vi "GetOpenChannels.vi"(7 "Slot":T1, 8 "Error In":errorcluster, 11 "Keithley 7001 In":refnum<visa-resource-name>) -> (0 "Error Out":errorcluster, 2 "Channels Opened?":bool[](array[boolean]), 3 "Keithley 7001 Out":refnum<visa-resource-name>)   [LabVIEW 2012, in "Keithley-7001.lvlib"]
uses:
  Keithley-7001.lvlib
  Controls/Slot.ctl
panel:
  # "33"
  # "34"
  # "35"
  # "1"
  # "2"
  # "3"
  # "4"
  # "5"
  # "6"
  # "7"
  # "8"
  # "9"
  # "10"
  # "11"
  # "12"
  # "13"
  # "14"
  # "15"
  # "16"
  # "17"
  # "18"
  # "19"
  # "20"
  # "21"
  # "22"
  # "23"
  # "24"
  # "25"
  # "26"
  # "27"
  # "28"
  # "29"
  # "30"
  # "31"
  # "32"
  # "36"
  # "37"
  # "38"
  # "39"
  # "40"
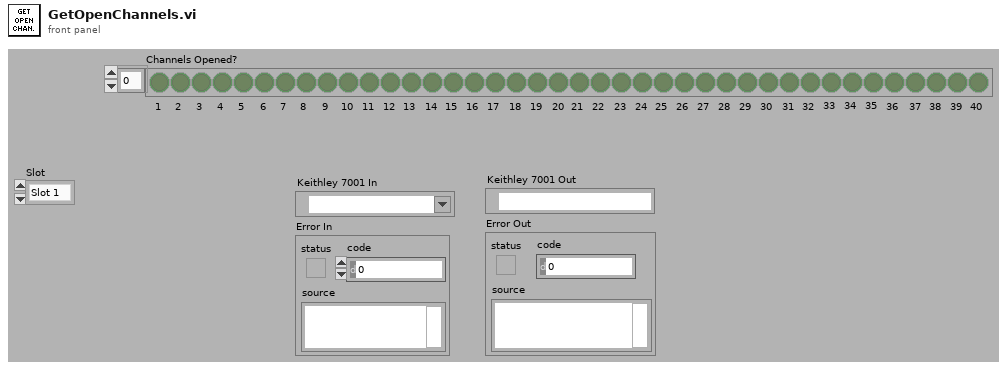
[diagram p1: front panel]
types:
  T1 = typedef "Keithley-7001.lvlib/Slot.ctl" = enum16{"Slot 1", "Slot 2"}
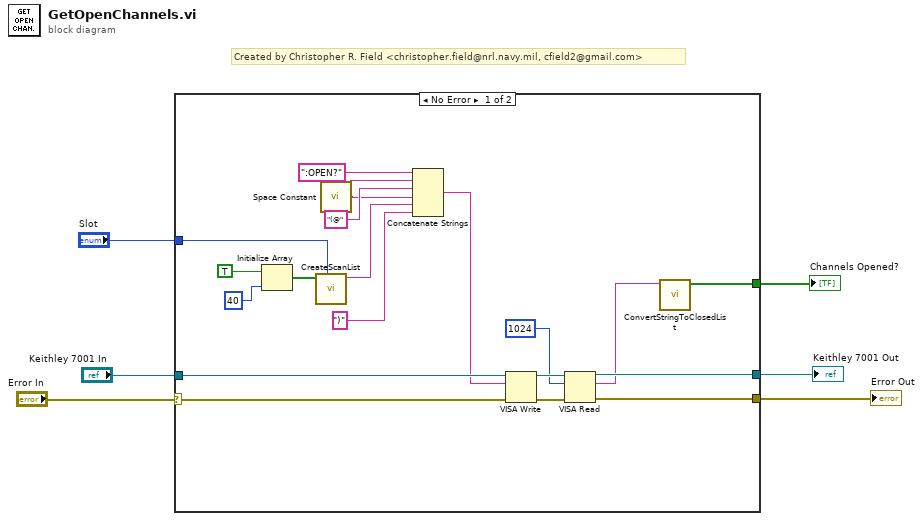
[diagram p0: block diagram]
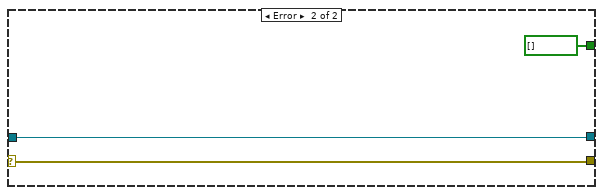
[diagram p2: hidden frame]
diagram:
  # "Created by Christopher R. Field <christopher.field@nrl.navy.mil, cfield2@gmail.com>"
  n1 = case shown="No Error" "Error In" {
    selector: "Error In" -> [w8 w28]
    tunnel: "Keithley 7001 In" -> [w23 w27]
    tunnel: [w22 w27] -> w5
    tunnel: [w21 w28] -> w4
    tunnel: [w12 bool[] [] ("Channels Closed?")] -> w3
    tunnel: "Slot" -> [w7 _]
    frame No Error {
      n2 = Initialize Array(TRUE, 40 ("dimension size")) -> (w9:bool[])
      n3 = call "CreateScanList.vi"("Slot"=w7, "Channels"=w9) -> ("Channel List"=w16:string)  [unwired: 9 in]
      n4 = call <vilib>:"Space Constant.vi"() -> ("String"=w17:string)
      n5 = Concatenate Strings(":OPEN?", w17, "(@", w17, w16, ")" ("string")) -> (w14:string)
      n6 = VISA Write(VISA resource name=w23, write buffer=w14, error in (no error)=w8) -> (VISA resource name out=w25:refnum<visa-resource-name>, error out=w24:errorcluster)  [unwired: 1 out]
      n7 = VISA Read(VISA resource name=w25, byte count=u32 1024, error in (no error)=w24) -> (VISA resource name out=w22:refnum<visa-resource-name>, read buffer=w13:string, error out=w21:errorcluster)  [unwired: 1 out]
      n8 = call "ConvertStringToClosedList.vi"("Channel List"=w13) -> ("Channels Closed"=w12:bool[])  [unwired: 10 in]
    }
    frame Error {
    }
  }
  "Keithley 7001 Out" <- w5
  "Error Out" <- w4
  "Channels Opened?" <- w3
